vi "Sets and Query the Limit for the Compare Function.vi"(5 "Enable to Query":bool=TRUE, 7 "Enable to Sets":bool=TRUE, 8 "error in":errorcluster, 9 "Upper Limit Value":dbl format="%#.6g", 10 "Lower Limit Value":dbl format="%#.6g", 11 "VISA resource name":refnum<visa-resource-name>) -> (0 "error out":errorcluster, 1 "Return the Upper Limit Value":string, 2 "Return the Lower Limit Value":string, 3 "VISA resource name out":refnum<visa-resource-name>)   [LabVIEW 2011, in "DMM4.lvlib"]
uses:
  <instrlib>/DMM4/DMM4.lvlib
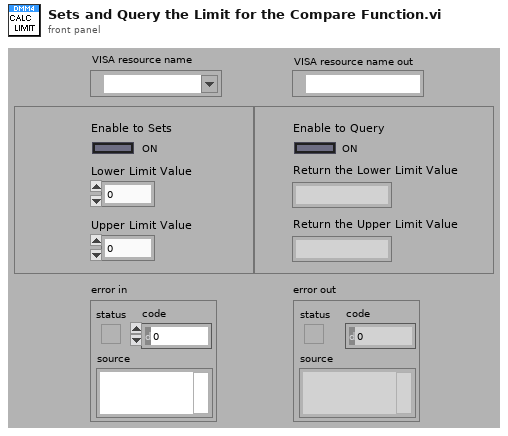
[diagram p1: front panel]
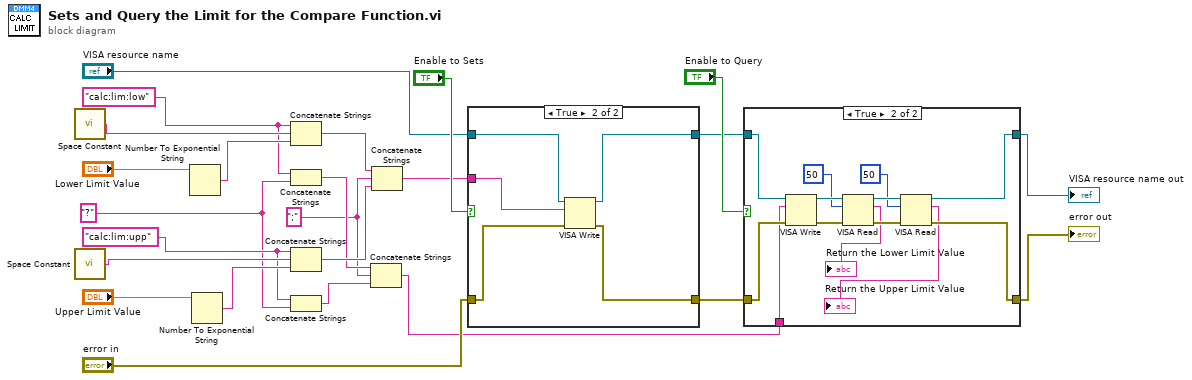
[diagram p0: block diagram]
diagram:
  w14 = ";" ("string")
  w18 = "?" ("string")
  w19 = "calc:lim:upp"
  w22 = "calc:lim:low"
  n1 = call <vilib>:"Space Constant.vi"() -> ("String"=w24:string)
  n2 = call <vilib>:"Space Constant.vi"() -> ("String"=w21:string)
  n3 = Number To Exponential String(number="Lower Limit Value") -> (E-format string=w23:string)  [unwired: 3 in]
  n4 = Number To Exponential String(number="Upper Limit Value") -> (E-format string=w20:string)  [unwired: 3 in]
  n5 = Concatenate Strings(w22, w24, w23) -> (w17:string)
  n6 = Concatenate Strings(w22, w18) -> (w15:string)
  n7 = Concatenate Strings(w19, w21, w20) -> (w16:string)
  n8 = Concatenate Strings(w19, w18) -> (w13:string)
  n9 = Concatenate Strings(w15, w14, w13) -> (w3:string)
  n10 = Concatenate Strings(w17, w14, w16) -> (w11:string)
  n11 = case shown="True" "Enable to Sets" {
    tunnel: w11 -> [_ w31]
    tunnel: "VISA resource name" -> [w26 w30]
    tunnel: "error in" -> [w25 w29]
    tunnel: [w26 w28] -> w7
    tunnel: [w25 w27] -> w6
    frame False {
    }
    frame True {
      n12 = VISA Write(VISA resource name=w30, write buffer=w31, error in (no error)=w29) -> (VISA resource name out=w28:refnum<visa-resource-name>, error out=w27:errorcluster)  [unwired: 1 out]
    }
  }
  n13 = case shown="True" "Enable to Query" {
    tunnel: w7 -> [w33 w40]
    tunnel: [w33 w38] -> w5
    tunnel: w6 -> [w32 w39]
    tunnel: [w32 w37] -> w4
    tunnel: w3 -> [_ w34]
    frame False {
    }
    frame True {
      n14 = VISA Write(VISA resource name=w40, write buffer=w34, error in (no error)=w39) -> (VISA resource name out=w45:refnum<visa-resource-name>, error out=w46:errorcluster)  [unwired: 1 out]
      n15 = VISA Read(VISA resource name=w45, byte count=u32 50, error in (no error)=w46) -> (VISA resource name out=w43:refnum<visa-resource-name>, read buffer=→"Return the Lower Limit Value":string, error out=w44:errorcluster)  [unwired: 1 out]
      n16 = VISA Read(VISA resource name=w43, byte count=u32 50, error in (no error)=w44) -> (VISA resource name out=w38:refnum<visa-resource-name>, read buffer=→"Return the Upper Limit Value":string, error out=w37:errorcluster)  [unwired: 1 out]
    }
  }
  "VISA resource name out" <- w5
  "error out" <- w4
